vi "Add WAMP-SCRAM authenticator.vi"(7 "Client Key":string, 8 "error in (no error)":errorcluster, 9 "Secret":string, 10 "Authentication ID":string, 11 "WAMP Client in":refnum<class "WAMP Client.lvclass">) -> (0 "error out":errorcluster, 3 "WAMP Client out":refnum<class "WAMP Client.lvclass">)   [LabVIEW 2020, in "wamplv.lvlib" / "WAMP Client.lvclass"]
uses:
  WAMP Client.lvclass
  Private/Authenticators/WampScramAuthenticator/WampScramAuthenticator.lvclass
  C:/local/wamplv/Private/Authenticators/IAuthenticator/IAuthenticator.lvclass
  WAMP Client.lvclass/WAMP Client.ctl
  C:/local/wamplv/Private/Authenticators/SecretBasedAuthenticatorBase/SecretBasedAuthenticatorBase.lvclass
  C:/local/wamplv/Private/Authenticators/WampScramAuthenticator/WampScramAuthenticator.lvclass
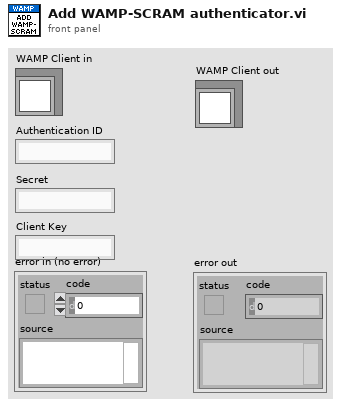
[diagram p1: front panel]
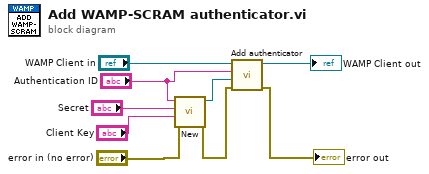
[diagram p0: block diagram]
diagram:
  n1 = call "New.vi"("error in (no error)"="error in (no error)", "Client Key"="Client Key", "Secret"="Secret", "Auth ID"="Authentication ID") -> ("error out"=w3:errorcluster, "WampScramAuthenticator"=w2:refnum<class "WampScramAuthenticator.lvclass">)  [unwired: 6 in]
  n2 = call "Add authenticator.vi"("error in (no error)"=w3, "IAuthenticator"=w2, "Authentication ID"="Authentication ID", "WAMP Client in"="WAMP Client in") -> ("error out"=→"error out":errorcluster, "WAMP Client out"=→"WAMP Client out":refnum<class "WAMP Client.lvclass">)  [unwired: 6 in]
